vi "Waveform graph.vi"() -> ()   [LabVIEW 2014]
doc: "Es VI te permite explorar de manera basica lo socntroles e indicadores de un programa en Labview."
panel:
  in  "Frequency":dbl(knob)=10.1 scale=0.0..10.0
  in  "Amplitude":dbl(knob)=10.0 scale=0.0..10.0
  out "Signal":dynamicdata(graph)
  in  "stop":bool
  # "Waveform Graph"
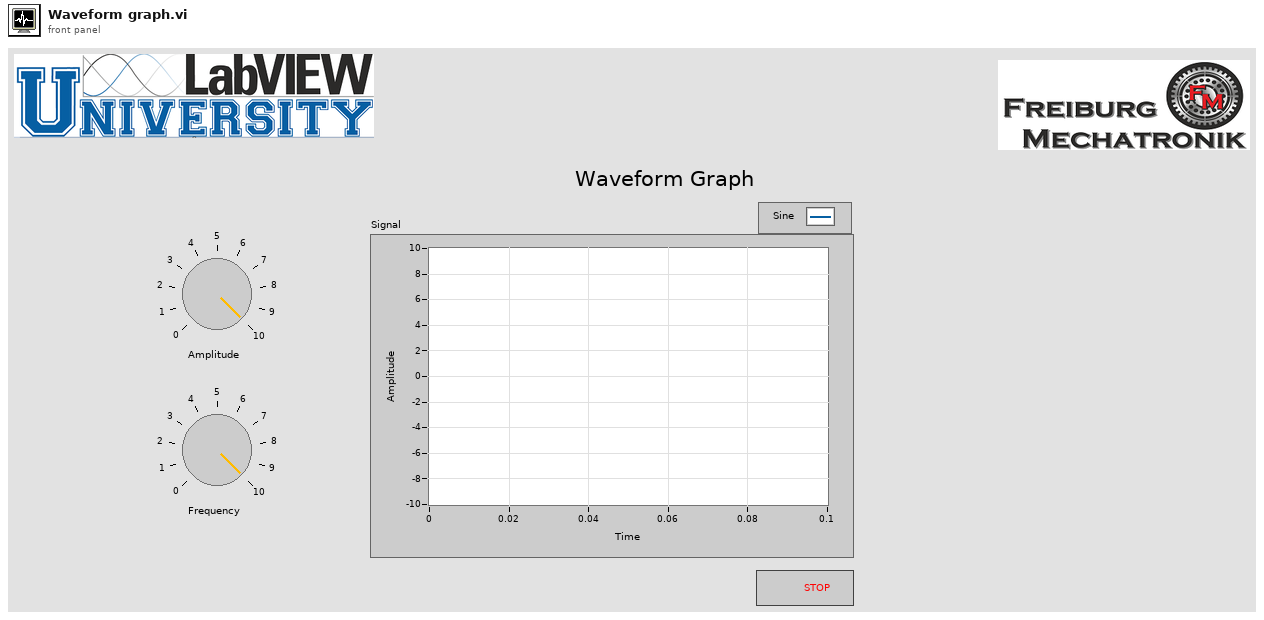
[diagram p1: front panel]
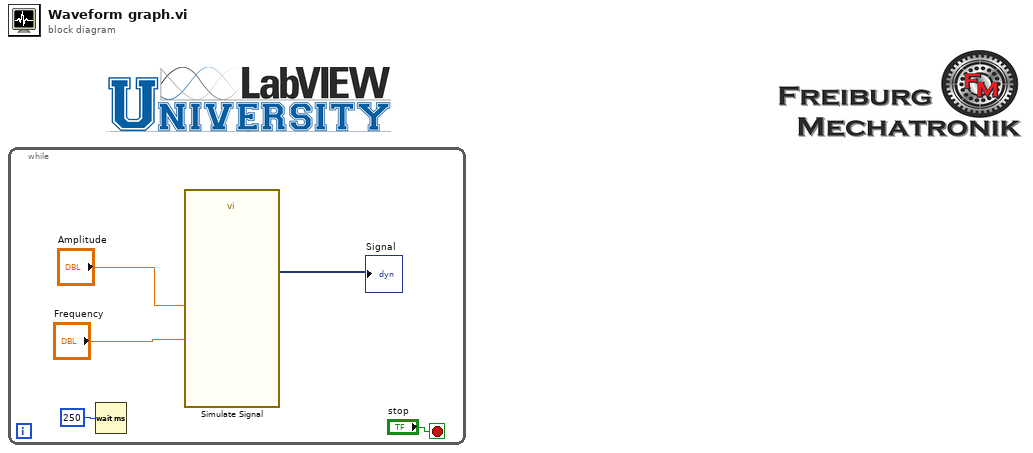
[diagram p0: block diagram]
diagram:
  n1 = while {
    stop <- "stop" stop-if-true
    n2 = Wait (ms)(milliseconds to wait=u32 250) -> ()  [unwired: 1 out]
    n3 = call "Simulate Signal"("Frequency"="Frequency", "Amplitude"="Amplitude") -> ("Sine"=→"Signal":dynamicdata)  [unwired: 12 in, 1 out]
  }
